vi "Read SerialSession.vi"(8 "error in (no error)":errorcluster, 11 "Meerstetter TEC in":refnum<class "Meerstetter TEC.lvclass">) -> (0 "error out":errorcluster, 2 "Session Handle":T1, 3 "Meerstetter TEC out":refnum<class "Meerstetter TEC.lvclass">)   [LabVIEW 2014, in "Meerstetter TEC.lvclass"]
uses:
  Meerstetter TEC.lvclass
  <userlib>/_Session Fwk/Typedefs/Session Handle.ctl
  <userlib>/_Session Fwk/Session - Root.lvclass
  Meerstetter TEC.lvclass/Meerstetter TEC.ctl
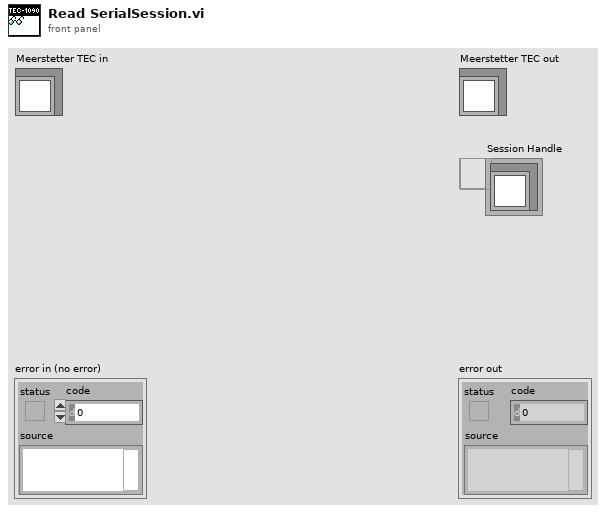
[diagram p1: front panel]
types:
  T1 = typedef "Session - Root.lvclass/Session Handle.ctl" = refnum<data-value>
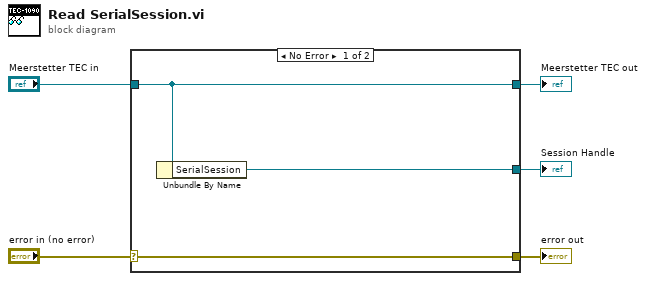
[diagram p0: block diagram]
diagram:
  n1 = case shown="No Error" "error in (no error)" {
    selector: "error in (no error)" -> [w8 w9]
    tunnel: [w8 w9] -> w4
    tunnel: [w7 w10] -> w2
    tunnel: "Meerstetter TEC in" -> [w7 w10]
    tunnel: [w6 _] -> w1
    frame No Error {
      n2 = Unbundle By Name(w7) -> ("SerialSession"=w6:T1)
    }
    frame Error {
    }
  }
  "error out" <- w4
  "Meerstetter TEC out" <- w2
  "Session Handle" <- w1
